vi "Logger-Init Log File.vi"(0 "Folder":path, 5 "Name":string, 11 "error in (no error)":errorcluster) -> (4 "File path":path, 15 "error out":errorcluster)   [LabVIEW 2020]
uses:
  Typedefs/Logger-Level.ctl
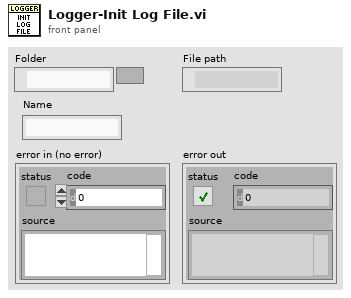
[diagram p1: front panel]
types:
  T1 = typedef "Logger-Level.ctl" = enum16{"Debug", "TCP", "Info", "Warning", "Error", "Critical"}
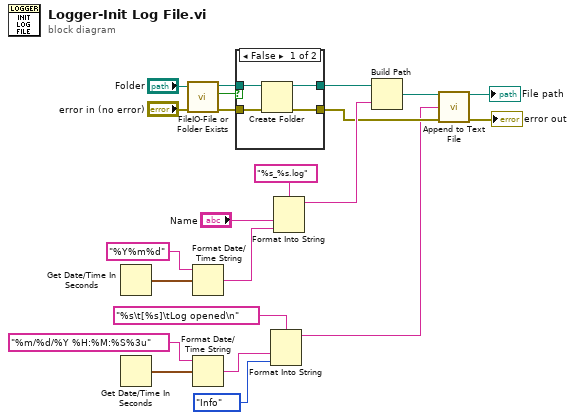
[diagram p0: block diagram]
diagram:
  n1 = Get Date/Time In Seconds() -> (seconds since 1Jan1904=w16:timestamp)
  n2 = Get Date/Time In Seconds() -> (seconds since 1Jan1904=w5:timestamp)
  n3 = call "FileIO-File or Folder Exists.vi"("error in (no error)"="error in (no error)", "path"="Folder") -> ("error out"=w18:errorcluster, "Directory?"=w19:bool, "dup path"=w20:path)  [unwired: 6 in, 1 out]
  n4 = Format Date/Time String(time format string (%c)="%Y%m%d", seconds (now)=w16) -> (date/time string=w13:string)  [unwired: 1 in]
  n5 = Format Date/Time String(time format string (%c)="%m/%d/%Y %H:%M:%S%3u", seconds (now)=w5) -> (date/time string=w2:string)  [unwired: 1 in]
  n6 = case shown="False" w19 {
    tunnel: w20 -> [w26 w28]
    tunnel: [w24 w28] -> w12
    tunnel: w18 -> [w25 w27]
    tunnel: [w23 w27] -> w9
    frame False {
      n7 = Create Folder(path (use dialog)=w26, error in=w25) -> (created path=w24:path, error out=w23:errorcluster)  [unwired: 1 in, 1 out]
    }
    frame True {
    }
  }
  n8 = Format Into String(format string="%s\t[%s]\tLog opened\n", w2, Logger-Level."Info" ("Level")) -> (resulting string=w3:string)  [unwired: 2 in, 1 out]
  n9 = Format Into String(format string="%s_%s.log", "Name", w13) -> (resulting string=w11:string)  [unwired: 2 in, 1 out]
  n10 = Build Path(base path=w12, name or relative path=w11) -> (appended path=w10:path)
  n11 = call "Append to Text File.vi"("file path"=w10, "text"=w3, "error in (no error)"=w9) -> ("file path out"=→"File path":path, "error out"=→"error out":errorcluster)  [unwired: 11 in]
